vi "Write Control Index.vi"(8 "error in (no error)":errorcluster, 10 "Control Index":i32, 11 "UI-Bus Control in":refnum<class "UI-Bus Control.lvclass">) -> (0 "error out":errorcluster, 3 "UI-Bus Control out":refnum<class "UI-Bus Control.lvclass">)   [LabVIEW 2021, in "UI-Bus Control.lvclass"]
uses:
  UI-Bus Control.lvclass
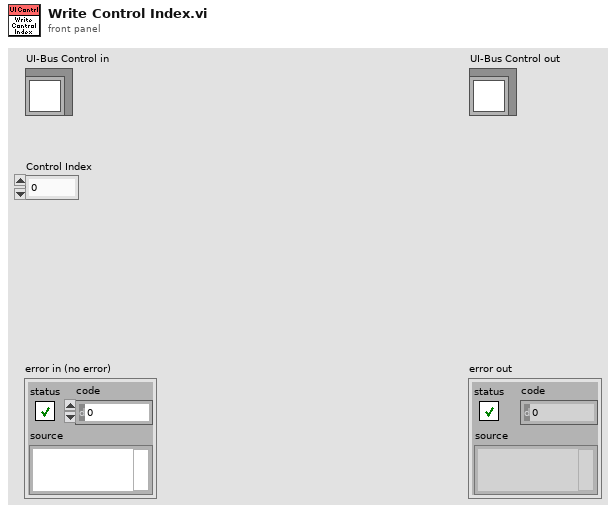
[diagram p1: front panel]
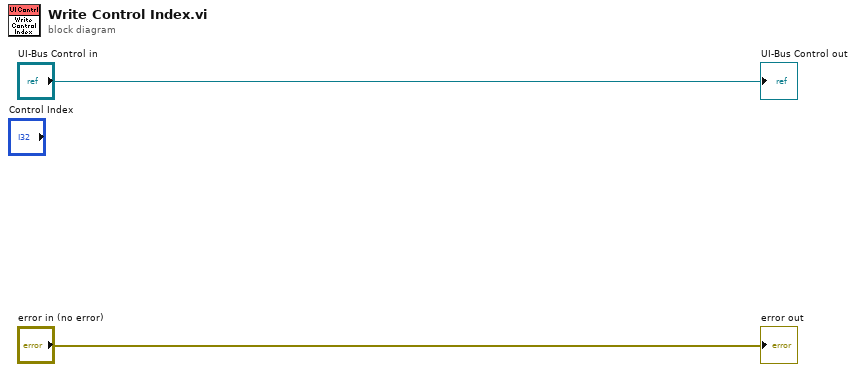
[diagram p0: block diagram]
diagram:
  "error out" <- "error in (no error)"
  "UI-Bus Control out" <- "UI-Bus Control in"
